vi "height name set.vi"(7 "height name":T1, 8 "error in (no error)":errorcluster, 9 "plus 2":bool, 11 "offset":dbl) -> (0 "error out":errorcluster)   [LabVIEW 2019]
uses:
  ctl/height.ctl
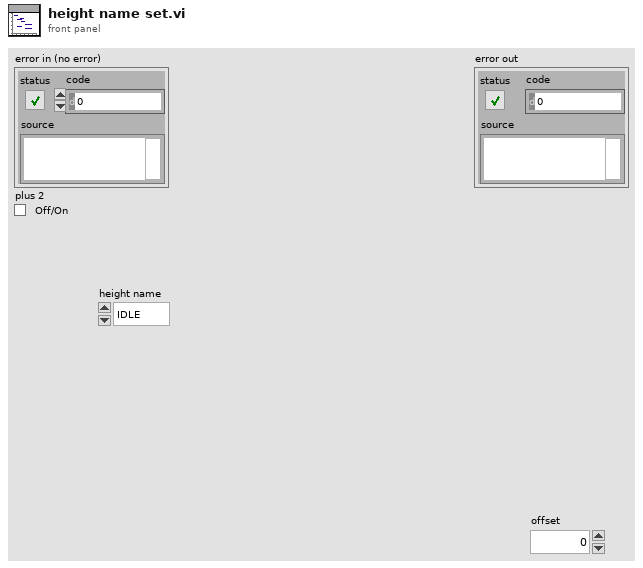
[diagram p1: front panel]
types:
  T1 = typedef "height.ctl" = enum16{"IDLE", "recycle pre-catch", "recycle catch", "recycle zone", "vision height", "box 1", "box 2", "box 3", "box 1 pre", "box 2 pre", "box 3 pre", "reg 1", "reg 2", "reg 1 pre", "reg 2 pre", "put 1", "put 2", "put 3"}
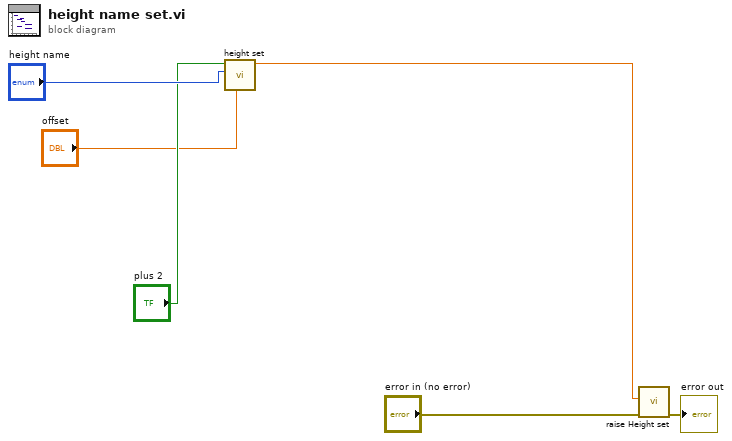
[diagram p0: block diagram]
diagram:
  n1 = call "height set.vi"("offset"="offset", "height name"="height name", "plus in"="plus 2") -> ("Numeric"=w3:dbl)  [unwired: 8 in]
  n2 = call "raise Height set.vi"("error in (no error)"="error in (no error)", "Height_cm"=w3) -> ("error out"=→"error out":errorcluster)  [unwired: 9 in]
